vi "solar_misc List StaticVIs.vi"(8 "error in (no error)":errorcluster, 11 "VI Refnum":refnum<vi>) -> (0 "error out":errorcluster, 2 "StaticVIs":string[](array[string]), 3 "dup VI Refnum":refnum<vi>)   [LabVIEW 2018]
doc: "This gets the static VI references loaded on the VI's block diagram. Useful for determining the SOLAR target's loaded in a SOLAR application."
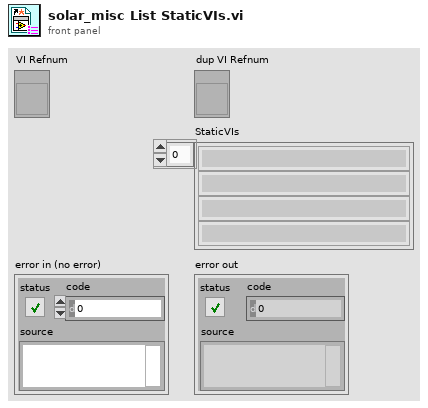
[diagram p1: front panel]
types:
  T1 = enum8{"Include the clone VI", "Include the original reentrant VI instead of the clone VI", "Include both the original reentrant VI and the clone VI"}
  T2 = enum8{"No dynamic dispatch VIs", "Include nearest implementation", "Include all overrides"}
  T3 = enum8{"Only include commented out diagrams if diagram already loaded", "Never include commented out diagrams", "Always include commented out diagrams"}
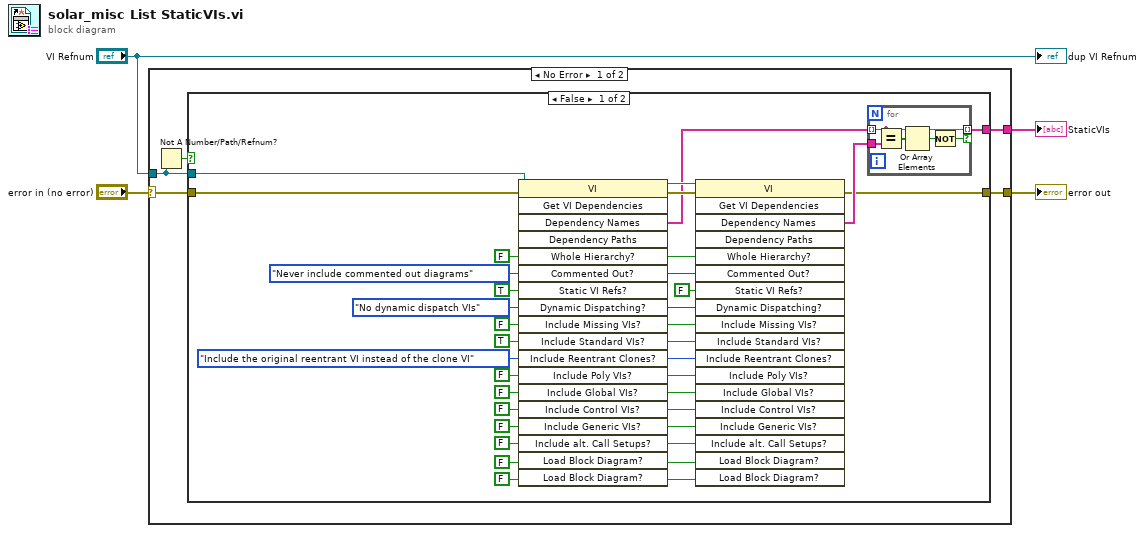
[diagram p0: block diagram]
diagram:
  n1 = case shown="No Error" "error in (no error)" {
    selector: "error in (no error)" -> [w9 w39]
    tunnel: "VI Refnum" -> [w6 _]
    tunnel: [w8 w39] -> w2
    tunnel: [w7 _] -> w1
    frame No Error {
      n2 = Not A Number/Path/Refnum?(number/path/refnum=w6) -> (NaN/Path/Refnum?=w5:bool)
      n3 = case shown="False" w5 {
        tunnel: w6 -> [w13 _]
        tunnel: w9 -> [w12 w38]
        tunnel: [w11 w38] -> w8
        tunnel: [w10 _] -> w7
        frame False {
          w19 = FALSE ("Load Block Diagram?")
          w20 = FALSE ("Keep Express VIs?")
          w21 = FALSE ("Include Alternate Call Setups?")
          w22 = FALSE ("Include Generic VIs?")
          w23 = FALSE ("Include Control VIs?")
          w24 = FALSE ("Include Global VIs?")
          w25 = FALSE ("Include Poly VIs?")
          w16 = T1."Include the original reentrant VI instead of the clone VI" ("Include Reentrant Clones?")
          w26 = TRUE ("Include Standard VIs?")
          w27 = FALSE ("Include Missing Items?")
          w28 = T2."No dynamic dispatch VIs" ("Dynamic Dispatching?")
          w17 = T3."Never include commented out diagrams" ("Commented Out Diagrams?")
          w29 = FALSE ("Whole Hierarchy?")
          n4 = invoke class="VI" method="Get VI Dependencies"(reference=w13, error in=w12, "Whole Hierarchy?"=w29, "Commented Out?"=w17, "Static VI Refs?"=TRUE, "Dynamic Dispatching?"=w28, "Include Missing VIs?"=w27, "Include Standard VIs?"=w26, "Include Reentrant Clones?"=w16, "Include Poly VIs?"=w25, "Include Global VIs?"=w24, "Include Control VIs?"=w23, "Include Generic VIs?"=w22, "Include alt. Call Setups?"=w21, "Load Block Diagram?"=w20, "Load Block Diagram?"=w19) -> (reference out=w30:refnum<vi>, error out=w31:errorcluster, "Dependency Names"=w15:string[])  [unwired: 3 in, 16 out]
          n5 = invoke class="VI" method="Get VI Dependencies"(reference=w30, error in=w31, "Whole Hierarchy?"=w29, "Commented Out?"=w17, "Static VI Refs?"=FALSE, "Dynamic Dispatching?"=w28, "Include Missing VIs?"=w27, "Include Standard VIs?"=w26, "Include Reentrant Clones?"=w16, "Include Poly VIs?"=w25, "Include Global VIs?"=w24, "Include Control VIs?"=w23, "Include Generic VIs?"=w22, "Include alt. Call Setups?"=w21, "Load Block Diagram?"=w20, "Load Block Diagram?"=w19) -> (error out=w11:errorcluster, "Dependency Names"=w14:string[])  [unwired: 3 in, 17 out]
          n6 = for {
            tunnel: w14 -> [w37]
            tunnel: w15 -> [w36] mode=indexing
            tunnel: [w36] -> w10 mode=indexing if=w33
            n7 = Equal?(x=w36, y=w37) -> (x = y?=w35:bool[])
            n8 = Or Array Elements(Boolean array=w35) -> (logical OR=w34:bool)
            n9 = Not(x=w34) -> (.not. x?=w33:bool)
          }
        }
        frame True {
        }
      }
    }
    frame Error {
    }
  }
  "error out" <- w2
  "StaticVIs" <- w1
  "dup VI Refnum" <- "VI Refnum"
